vi "TCPwrite512B-client.vi"(8 "Error in":errorcluster, 10 "Cmd In":string, 11 "connection ID in":refnum<k5>) -> (0 "Error out":errorcluster, 3 "connection ID out":refnum<k5>)   [LabVIEW 2013]
panel:
  out "bytes written":i32
  out "TCP receiving time":u32
  out "TCP time in":u32
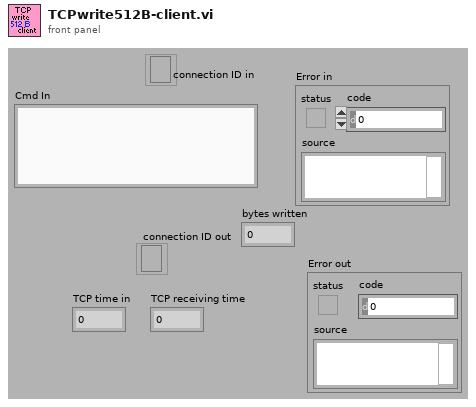
[diagram p1: front panel]
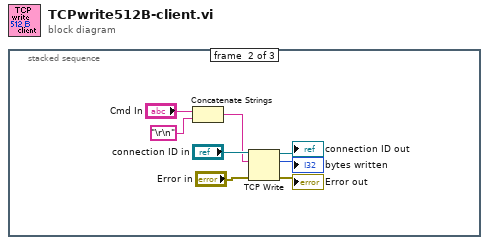
[diagram p0: block diagram]
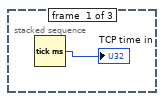
[diagram p2: hidden frame]
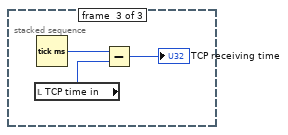
[diagram p3: hidden frame]
diagram:
  n1 = stacked-sequence {
    frame #0 {
      n2 = Tick Count (ms)() -> (millisecond timer value=→"TCP time in":u32)
    }
    frame #1 {
      n3 = Concatenate Strings("Cmd In", "\r\n") -> (w3:string)
      n4 = TCP Write(connection ID="connection ID in", data in=w3, error in (no error)="Error in") -> (connection ID out=→"connection ID out":refnum<k5>, bytes written=→"bytes written":i32, error out=→"Error out":errorcluster)  [unwired: 1 out]
    }
    frame #2 {
      n5 = local read "TCP time in"() -> (w10:u32)
      n6 = Tick Count (ms)() -> (millisecond timer value=w12:u32)
      n7 = Subtract(x=w12, y=w10) -> (x-y=→"TCP receiving time":u32)
    }
  }
